vi "Main.vi"(11 "error in (no error)":errorcluster) -> (15 "error out":errorcluster)   [LabVIEW 2021]
uses:
  Controls/Operation.ctl
  Controls/State Cluster.ctl
  Controls/Main Data Cluster.ctl
  Classes/Sender/Sender UI.vi
  Classes/Sender/Sender.lvclass
  Classes/Receiver/Receiver UI.vi
  Classes/Receiver/Receiver.lvclass
  Controls/User Event Operation.ctl
  Downloads/Sample PC Template/Sample PC Template/Typedefs/Data.ctl
  Downloads/Sample PC Template/Sample PC Template/Sample PC Template.lvlib
panel:
  in  "Load Receiver":bool
  in  "Load Sender":bool
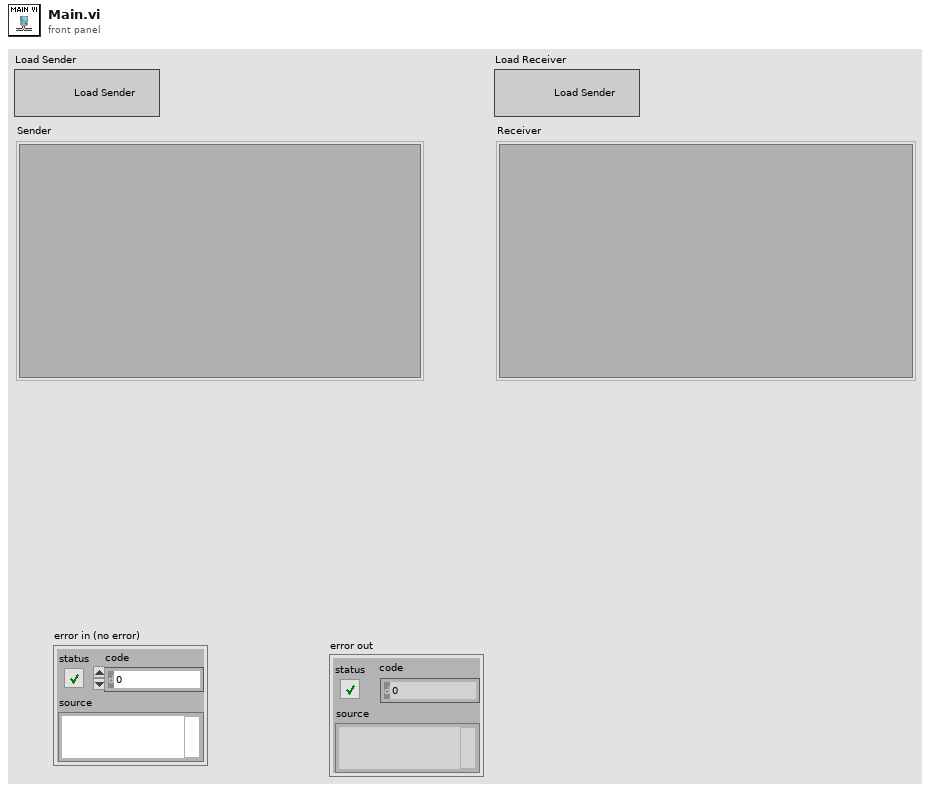
[diagram p1: front panel]
types:
  T1 = typedef "Main Data Cluster.ctl" = cluster{"user event out":refnum<user-event>}
  T2 = typedef "State Cluster.ctl" = cluster{"State":string, "Data":variant}
  T3 = typedef "Operation.ctl" = enum16{"Create", "Enqueue", "Enqueue N", "Enstack", "Dequeue", "Flush", "Release"}
  T4 = typedef "Sample PC Template.lvlib/Data.ctl" = cluster{"State":string, "Data":variant}
  T5 = typedef "User Event Operation.ctl" = enum16{"Obtain", "Generate", "Release"}
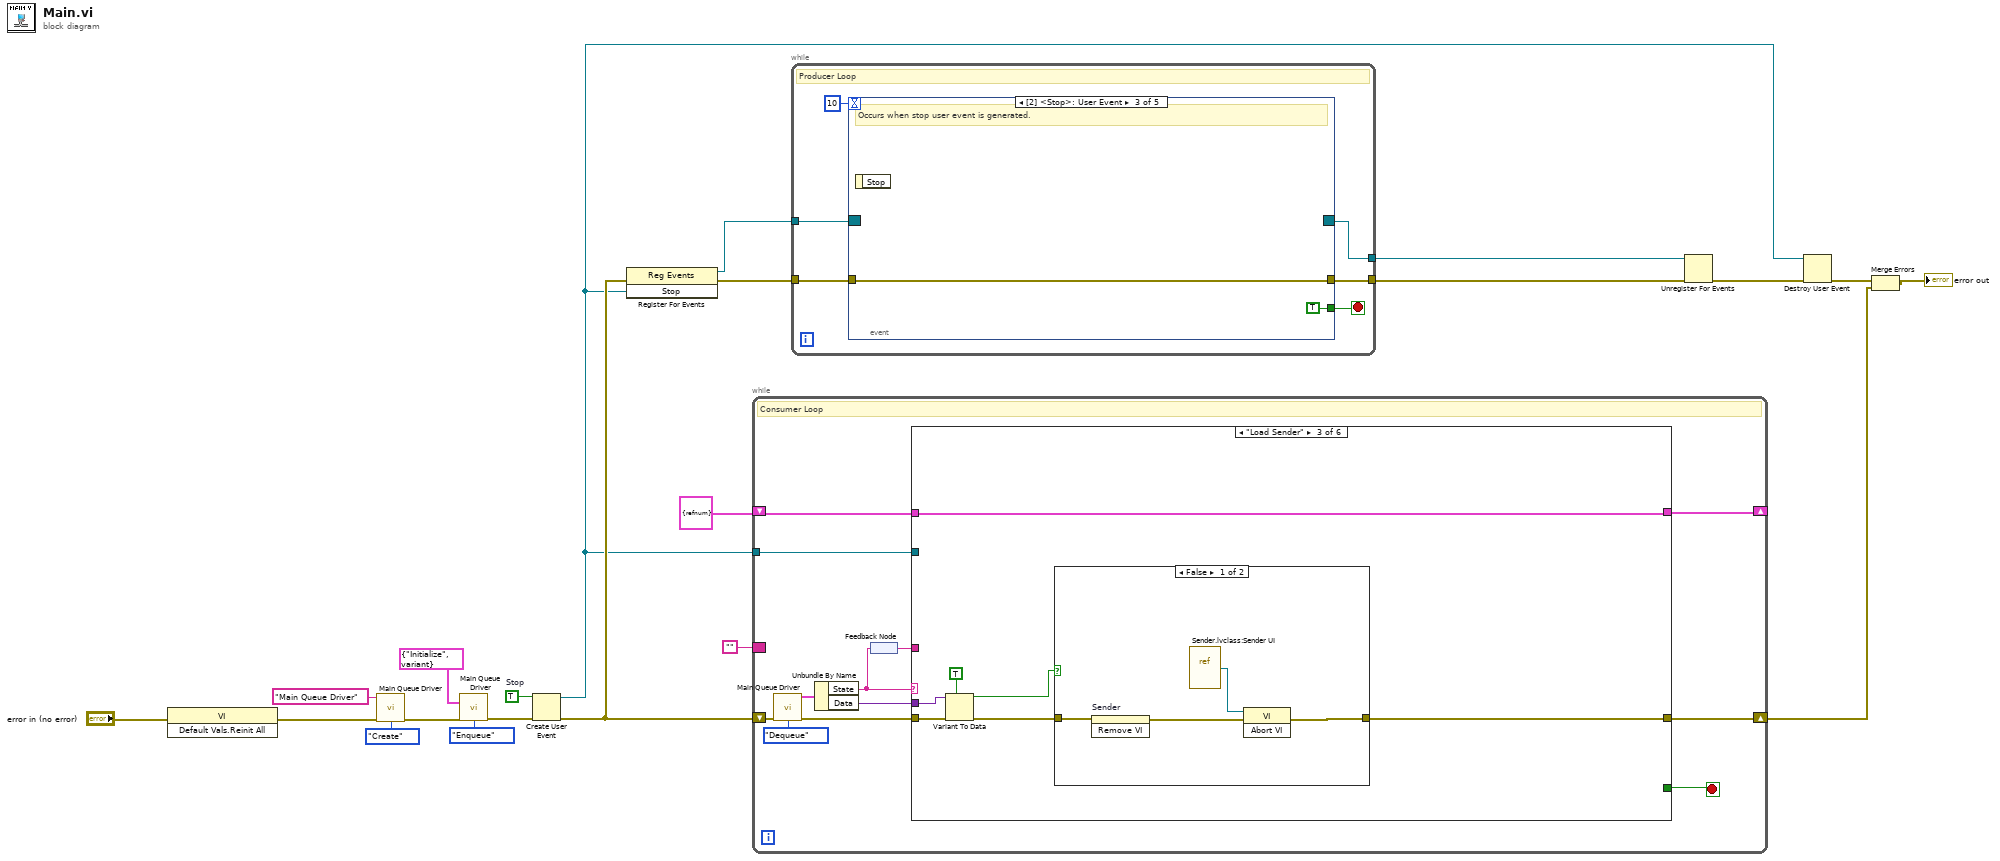
[diagram p0: block diagram]
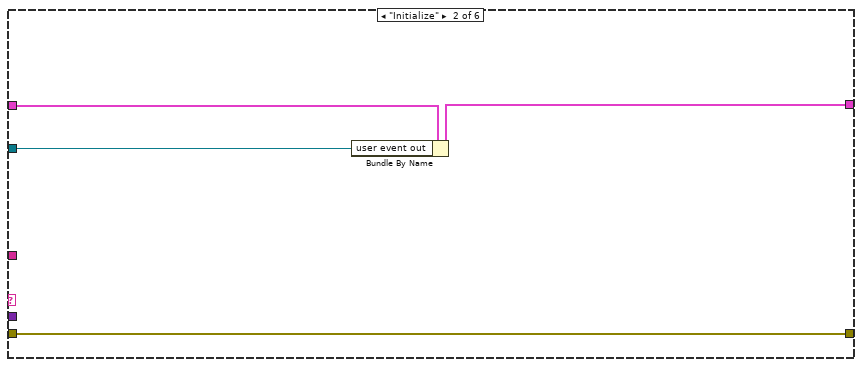
[diagram p3: hidden frame]
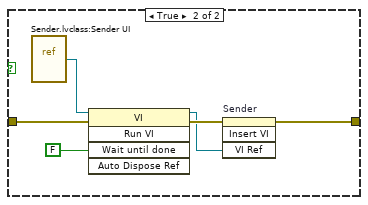
[diagram p4: hidden frame]
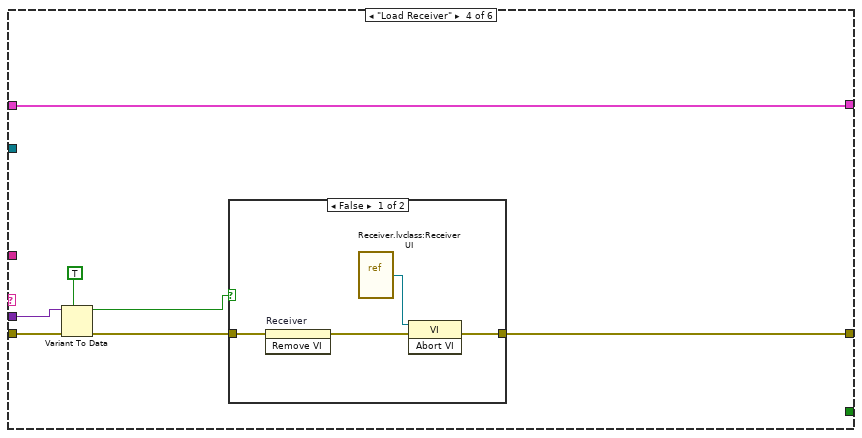
[diagram p5: hidden frame]
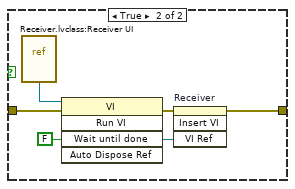
[diagram p6: hidden frame]
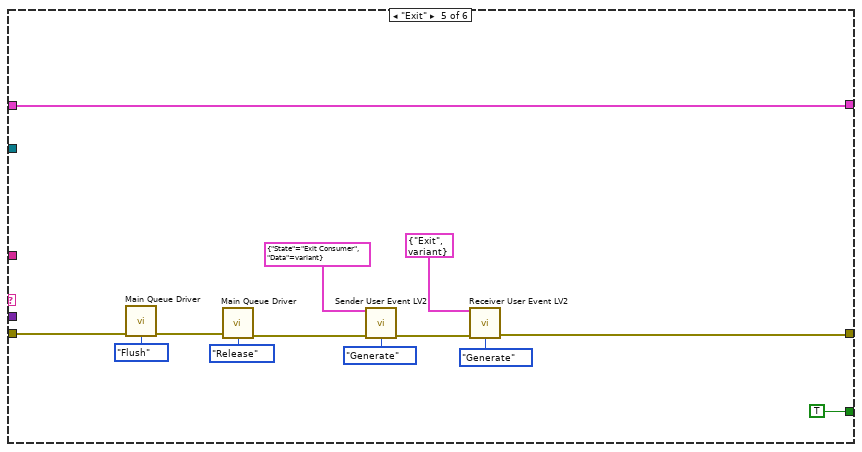
[diagram p7: hidden frame]
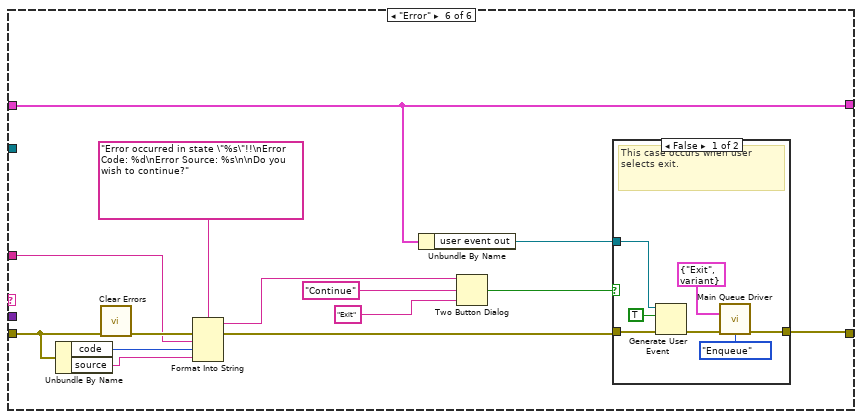
[diagram p8: hidden frame]
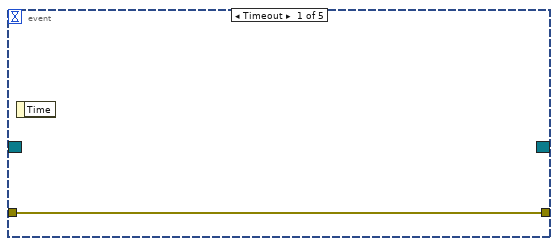
[diagram p10: hidden frame]
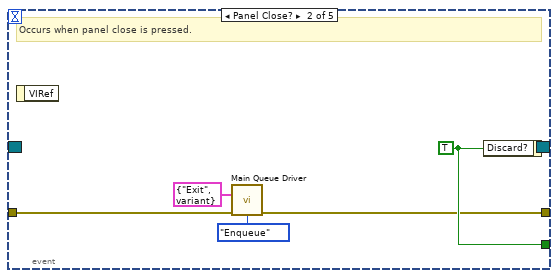
[diagram p11: hidden frame]
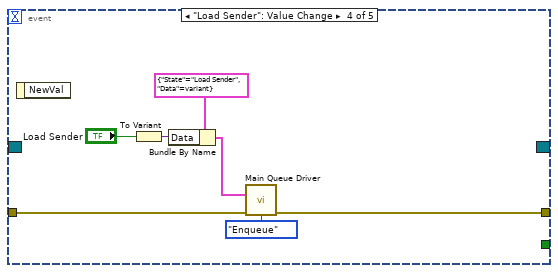
[diagram p12: hidden frame]
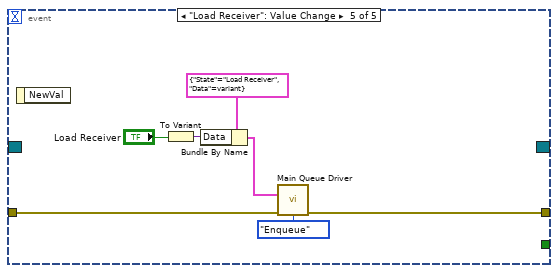
[diagram p13: hidden frame]
diagram:
  w15 = TRUE  # Stop
  n1 = invoke class="VI" method="Default Vals.Reinit All"(error in="error in (no error)") -> (error out=w1:errorcluster)  [unwired: 2 in, 2 out]
  n2 = call "Main Queue Driver.vi"("Queue Name"="Main Queue Driver", "error in (no error)"=w1, "Operations"=Operation."Create") -> ("error out"=w19:errorcluster)  [unwired: 11 in, 1 out]
  n3 = call "Main Queue Driver.vi"("State"=T2 {"State"="Initialize", "Data"=variant}, "error in (no error)"=w19, "Operations"=Operation."Enqueue") -> ("error out"=w16:errorcluster)  [unwired: 11 in, 1 out]
  n4 = Create User Event(user event datatype=w15, error in=w16) -> (user event=w3:refnum<user-event>, error out=w14:errorcluster)
  n5 = register-events(error in=w14, w3) -> (reference out=w12:refnum<event-registration>, error out=w13:errorcluster)  [unwired: 1 in]
  n6 = while {
    shift-right: [w27] -> w6
    shift-left: w14 -> [w32]
    border: "" -> [_]
    tunnel: w3 -> [w24]
    shift-right: [w23] -> _
    shift-left: T1 {"user event out"=refnum} -> [w25]
    stop <- w26 stop-if-true
    # "Consumer Loop"
    n7 = call "Main Queue Driver.vi"("error in (no error)"=w32, "Operations"=Operation."Dequeue") -> ("Dequeued Element"=w30:T2, "error out"=w31:errorcluster)  [unwired: 12 in]
    n8 = Unbundle By Name(w30) -> ("State"=w28:string, "Data"=w29:variant)
    n9 = feedback-in #1(w28) -> ()
    n10 = feedback #1() -> (w22:string)
    n11 = case shown="\"Load Sender\"" w28 {
      tunnel: w31 -> [w35 w36 w45 w62 w85 w93]
      tunnel: w29 -> [_ _ w42 w59 _ _]
      tunnel: [w35 w36 w44 w61 w78 w90] -> w27
      tunnel: [_ _ _ _ TRUE _] -> w26
      tunnel: w25 -> [w34 w39 w46 w63 w81 w89]
      tunnel: w24 -> [_ w38 _ _ _ _]
      tunnel: [w34 w37 w46 w63 w81 w89] -> w23
      tunnel: w22 -> [_ _ _ _ _ w87]
      frame Default {
      }
      frame "Initialize" {
        n12 = Bundle By Name(cluster=w39, "user event out"=w38) -> (w37:T1)
      }
      frame "Load Sender" {
        n13 = Variant To Data(error in=w45, type=TRUE, Variant=w42) -> (data=w40:bool, error out=w43:errorcluster)
        n14 = case shown="False" w40 {
          tunnel: [w47 w56] -> w44
          tunnel: w43 -> [w49 w55]
          frame False {
            n15 = invoke on="Sender" class="SubPnl" method="Remove VI"(error in=w49) -> (error out=w48:errorcluster)  [unwired: 2 in, 2 out]
            n16 = vi-ref "Sender.lvclass:Sender UI.vi"() -> (w50:refnum<vi>)
            n17 = invoke class="VI" method="Abort VI"(reference=w50, error in=w48) -> (error out=w47:errorcluster)  [unwired: 1 in, 2 out]
          }
          frame True {
            n18 = vi-ref "Sender.lvclass:Sender UI.vi"() -> (w53:refnum<vi>)
            n19 = invoke class="VI" method="Run VI"(reference=w53, error in=w55, "Wait until done"=FALSE ("Wait Until Done")) -> (reference out=w51:refnum<vi>, error out=w54:errorcluster)  [unwired: 2 in, 3 out]
            n20 = invoke on="Sender" class="SubPnl" method="Insert VI"(error in=w54, "VI Ref"=w51) -> (error out=w56:errorcluster)  [unwired: 2 in, 3 out]
          }
        }
      }
      frame "Load Receiver" {
        n21 = Variant To Data(error in=w62, type=TRUE, Variant=w59) -> (data=w57:bool, error out=w60:errorcluster)
        n22 = case shown="False" w57 {
          tunnel: [w64 w73] -> w61
          tunnel: w60 -> [w67 w72]
          frame False {
            n23 = invoke on="Receiver" class="SubPnl" method="Remove VI"(error in=w67) -> (error out=w65:errorcluster)  [unwired: 2 in, 2 out]
            n24 = vi-ref "Receiver.lvclass:Receiver UI.vi"() -> (w66:refnum<vi>)
            n25 = invoke class="VI" method="Abort VI"(reference=w66, error in=w65) -> (error out=w64:errorcluster)  [unwired: 1 in, 2 out]
          }
          frame True {
            n26 = vi-ref "Receiver.lvclass:Receiver UI.vi"() -> (w70:refnum<vi>)
            n27 = invoke class="VI" method="Run VI"(reference=w70, error in=w72, "Wait until done"=FALSE ("Wait Until Done")) -> (reference out=w69:refnum<vi>, error out=w71:errorcluster)  [unwired: 2 in, 3 out]
            n28 = invoke on="Receiver" class="SubPnl" method="Insert VI"(error in=w71, "VI Ref"=w69) -> (error out=w73:errorcluster)  [unwired: 2 in, 3 out]
          }
        }
      }
      frame "Exit" {
        n29 = call "Main Queue Driver.vi"("error in (no error)"=w85, "Operations"=Operation."Flush") -> ("error out"=w83:errorcluster)  [unwired: 12 in, 1 out]
        n30 = call "Main Queue Driver.vi"("error in (no error)"=w83, "Operations"=Operation."Release") -> ("error out"=w80:errorcluster)  [unwired: 12 in, 1 out]
        n31 = call "Sender User Event LV2.vi"("Data"=T4 {"State"="Exit Consumer", "Data"=variant}, "Error In"=w80, "Operation"=User_Event_Operation."Generate") -> ("Error Out"=w79:errorcluster)  [unwired: 11 in, 1 out]
        n32 = call "Receiver User Event LV2.vi"("Data"=T4 {"State"="Exit", "Data"=variant}, "Error In"=w79, "Operation"=User_Event_Operation."Generate") -> ("Error Out"=w78:errorcluster)  [unwired: 11 in, 1 out]
      }
      frame "Error" {
        n33 = Unbundle By Name(w93) -> ("code"=w92:i32, "source"=w91:string)
        n34 = call <vilib>:"Clear Errors.vi"("error in (no error)"=w93) -> ("error out"=w100:errorcluster)  [unwired: 5 in, 1 out]
        n35 = Format Into String(format string="Error occurred in state \"%s\"!!\nError Code: %d\nError Source: %s\n\nDo you wish to continue?", error in=w100, w87, w92, w91) -> (resulting string=w98:string, error out=w95:errorcluster)  [unwired: 1 in]
        n36 = Unbundle By Name(w89) -> ("user event out"=w88:refnum<user-event>)
        n37 = Two Button Dialog(message=w98, 1:"Exit" ("F button name (\"Cancel\")"), 2:"Continue" ("T button name (\"OK\")")) -> (T button?=w94:bool)
        n38 = case shown="False" w94 {
          tunnel: w95 -> [w107 w108]
          tunnel: [w103 w108] -> w90
          tunnel: w88 -> [w105 _]
          frame False {
            # "This case occurs when user selects exit."
            n39 = Generate User Event(user event=w105, event data cluster=TRUE ("event data"), error in=w107) -> (error out=w104:errorcluster)  [unwired: 1 in, 1 out]
            n40 = call "Main Queue Driver.vi"("State"=T2 {"State"="Exit", "Data"=variant}, "error in (no error)"=w104, "Operations"=Operation."Enqueue") -> ("error out"=w103:errorcluster)  [unwired: 11 in, 1 out]
          }
          frame True {
            # "This case occurs when user selects to continue."
          }
        }
      }
    }
  }
  n41 = while {
    tunnel: w13 -> [w113]
    tunnel: w12 -> [w112]
    tunnel: [w111] -> w10
    tunnel: [w110] -> w9
    stop <- w109 stop-if-true
    # "Producer Loop"
    n42 = event shown="[2] <Stop>: User Event" {
      selector: w112 -> [_ _ _ _ _]
      dyn-events: [_ _ _ _ _] -> w111
      timeout: 10 -> [_ _ _ _ _]
      tunnel: w113 -> [w115 w119 w122 w129 w132]
      tunnel: [w115 w118 w122 w128 w131] -> w110
      tunnel: [_ w120 TRUE ("Discard?") _ _] -> w109
      event Timeout {
        n43 = event-data() -> ()  [unwired: 1 in, 1 out]
      }
      event Panel Close? {
        w120 = TRUE ("Discard?")
        # "Occurs when panel close is pressed."
        n44 = event-data() -> ()  [unwired: 1 in, 1 out]
        n45 = call "Main Queue Driver.vi"("State"=T2 {"State"="Exit", "Data"=variant}, "error in (no error)"=w119, "Operations"=Operation."Enqueue") -> ("error out"=w118:errorcluster)  [unwired: 11 in, 1 out]
        n46 = event-data("Discard?"=w120) -> ()  [unwired: 1 in, 1 out]
      }
      event User Event {
        # "Occurs when stop user event is generated."
        n47 = event-data() -> ()  [unwired: 1 in, 1 out]
      }
      event "Load Sender": Value Change {
        n48 = event-data() -> ()  [unwired: 1 in, 1 out]
        n49 = To Variant(anything="Load Sender") -> (Variant=w125:variant)
        n50 = Bundle By Name(cluster=T2 {"State"="Load Sender", "Data"=variant} ("State"), "Data"=w125) -> (w123:T2)
        n51 = call "Main Queue Driver.vi"("State"=w123, "error in (no error)"=w129, "Operations"=Operation."Enqueue") -> ("error out"=w128:errorcluster)  [unwired: 11 in, 1 out]
      }
      event "Load Receiver": Value Change {
        n52 = event-data() -> ()  [unwired: 1 in, 1 out]
        n53 = To Variant(anything="Load Receiver") -> (Variant=w134:variant)
        n54 = Bundle By Name(cluster=T2 {"State"="Load Receiver", "Data"=variant} ("State"), "Data"=w134) -> (w133:T2)
        n55 = call "Main Queue Driver.vi"("State"=w133, "error in (no error)"=w132, "Operations"=Operation."Enqueue") -> ("error out"=w131:errorcluster)  [unwired: 11 in, 1 out]
      }
    }
  }
  n56 = Unregister For Events(event registration refnum=w10, error in=w9) -> (error out=w8:errorcluster)
  n57 = Destroy User Event(user event=w3, error in=w8) -> (error out=w7:errorcluster)
  n58 = Merge Errors(w7, w6) -> (→"error out":errorcluster)
